vi "ZCAN_ReadChannelErrInfo.vi"(1 "can_index_handle":u32, 3 "error in (no error)":errorcluster caption="错误输入（无错误）") -> (6 "ChannelErrInfo(string out)":string, 8 "error out":errorcluster caption="错误输出")   [LabVIEW 2013]
doc: "该函数用于读取通道的错误信息。"
uses:
  data_type/ZCAN_CHANNEL_ERROR_INFO.ctl
panel:
  in  "ZCAN_CHANNEL_ERROR_INFO(in)":T1
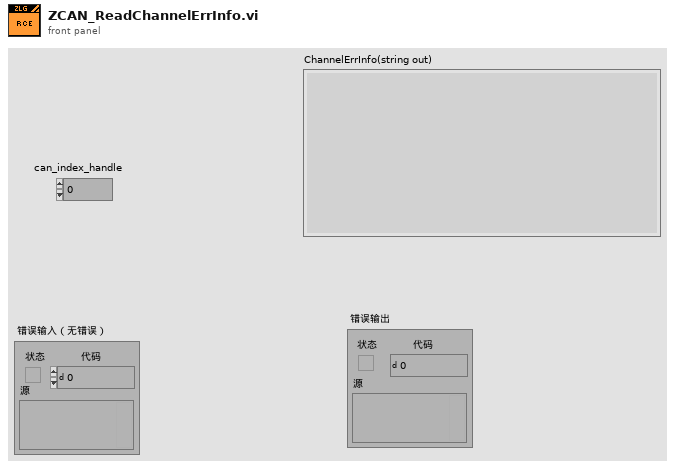
[diagram p1: front panel]
types:
  T1 = typedef "ZCAN_CHANNEL_ERROR_INFO.ctl" = cluster{"error_code":u32, "passive_ErrData":cluster{"byte0":u8, "byte1":u8, "byte3":u8}, "arLost_ErrData":u8}
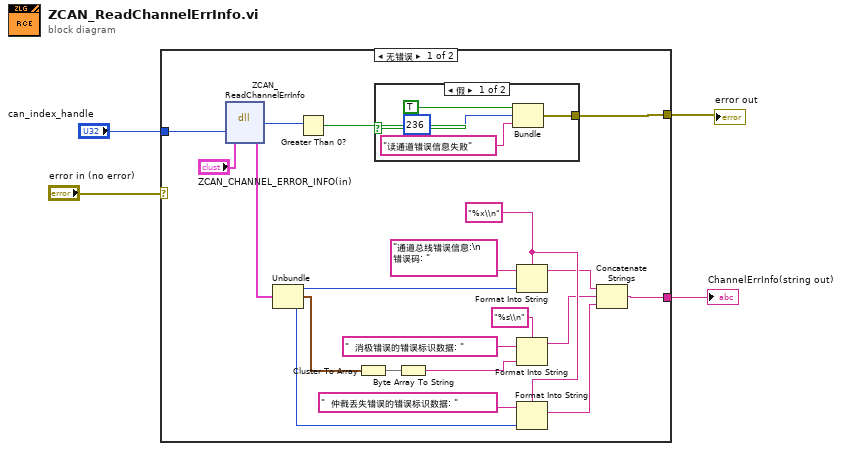
[diagram p0: block diagram]
diagram:
  n1 = case shown="无错误" "error in (no error)" {
    selector: "error in (no error)" -> [_ w29]
    tunnel: [w21 w29] -> w2
    tunnel: "can_index_handle" -> [w24 _]
    tunnel: [w10 _] -> w1
    frame No Error {
      w11 = "%x\\n" ("format string")
      n2 = dll-call lib="PTH1Jabs CUserschenhuachunDesktopUSBCAN-I系列binzlgcan_wrap.dll" fn="ZCAN_ReadChannelErrInfo"("channel_handle"=w24, "pErrInfo"="ZCAN_CHANNEL_ERROR_INFO(in)") -> ("return"=w23:u32, "pErrInfo"=w19:T1)  [unwired: 4 in, 2 out]
      n3 = Unbundle(w19) -> ("error_code"=w12:u32, "passive_ErrData"=w15:cluster{"byte0":u8, "byte1":u8, "byte3":u8}, "arLost_ErrData"=w7:u8)
      n4 = Greater Than 0?(x=w23) -> (x > 0?=w22:bool)
      n5 = Cluster To Array(cluster=w15) -> (array=w14:u8[])
      n6 = case shown="假" w22 {
        tunnel: [w25 _] -> w21
        frame False {
          n7 = Bundle("status"=TRUE, "code"=236, "消息"="读通道错误信息失败") -> (w25:cluster{"status":bool, "code":i32, "消息":string})  [unwired: 1 in]
        }
        frame True {
        }
      }
      n8 = Byte Array To String(unsigned byte array=w14) -> (string=w13:string)
      n9 = Format Into String(format string=w11, initial string="通道总线错误信息:\n  错误码: ", w12) -> (resulting string=w9:string)  [unwired: 1 in, 1 out]
      n10 = Format Into String(format string="%s\\n", initial string="  消极错误的错误标识数据: ", w13) -> (resulting string=w8:string)  [unwired: 1 in, 1 out]
      n11 = Format Into String(format string=w11, initial string="  仲裁丢失错误的错误标识数据: ", w7) -> (resulting string=w6:string)  [unwired: 1 in, 1 out]
      n12 = Concatenate Strings(w9, w8, w6) -> (w10:string)
    }
    frame Error {
    }
  }
  "error out" <- w2
  "ChannelErrInfo(string out)" <- w1
